vi "Change State.vi"(8 "error in (no error)":errorcluster, 10 "Target State Actor in":refnum<class "State Actor.lvclass">, 11 "State Actor in":refnum<class "State Actor.lvclass">) -> (0 "error out":errorcluster, 3 "State Actor out":refnum<class "State Actor.lvclass">)   [LabVIEW 2024, in "State Actor.lvlib" / "State Actor.lvclass"]
uses:
  State Actor.lvclass
  State Actor.lvclass/State Actor.ctl
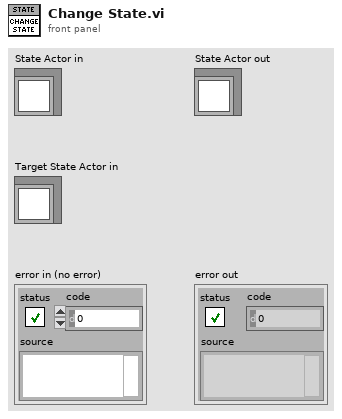
[diagram p1: front panel]
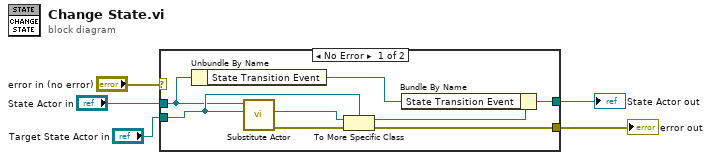
[diagram p0: block diagram]
diagram:
  n1 = case shown="No Error" "error in (no error)" {
    selector: "error in (no error)" -> [_ w15]
    tunnel: [w11 w15] -> w4
    tunnel: [w6 w14] -> w2
    tunnel: "State Actor in" -> [w9 w14]
    tunnel: "Target State Actor in" -> [w12 _]
    frame No Error {
      n2 = Unbundle By Name(w9) -> ("State Transition Event"=w7:refnum<user-event>)
      n3 = call-dynamic "Substitute Actor.vi"("Substitute Actor in"=w12, "Current Actor"=w9) -> ("error out"=w10:errorcluster, "Substitute Actor out"=w13:refnum<class "Actor.lvclass">)  [unwired: 8 in]
      n4 = To More Specific Class(target class=w12, reference=w13, error in=w10) -> (specific class reference=w8:refnum<class "State Actor.lvclass">, error out=w11:errorcluster)
      n5 = Bundle By Name(cluster=w8, "State Transition Event"=w7) -> (w6:refnum<class "State Actor.lvclass">)
    }
    frame Error {
    }
  }
  "error out" <- w4
  "State Actor out" <- w2
